vi "hFilterReg2014.vi"(4 "error in":errorcluster, 5 "Filter Modus":u16 format="%x", 6 "Frequenz":u16 format="%x", 7 "FPGA VI Reference In":refnum<k20>) -> (0 "error out":errorcluster, 2 "Timed Out":bool, 3 "FPGA VI Reference Out":refnum<k20>)   [LabVIEW 2014]
doc: "Schreibt eine gemeinsame Konfiguration in alle Filterregister."
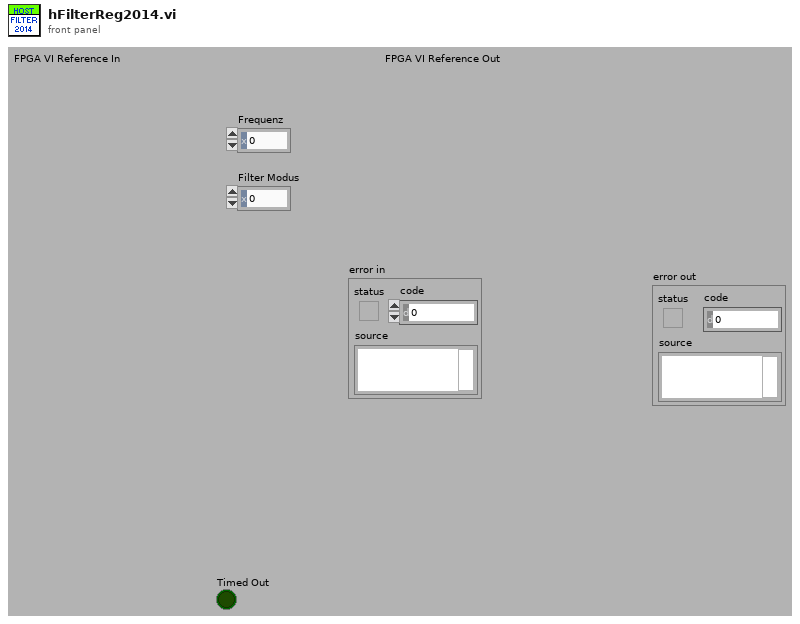
[diagram p1: front panel]
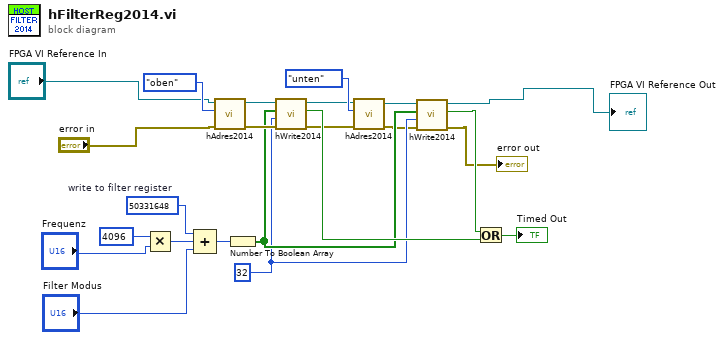
[diagram p0: block diagram]
diagram:
  w20 = u32 50331648  # write to filter register
  w6 = u8 32
  n1 = Multiply(x=u32 4096, y="Frequenz") -> (x*y=w21:u32)
  n2 = Compound Arithmetic op=ADD(w20, w21, "Filter Modus") -> (w22:u32)
  n3 = call "hAdres2014.vi"("error in"="error in", "AdressMode"=enum16{"select", "oben", "unten", "keinen"}."oben", "FPGA VI Reference In"="FPGA VI Reference In") -> ("error out"=w12:errorcluster, "FPGA VI Reference Out"=w13:refnum<k20>)  [unwired: 3 in]
  n4 = Number To Boolean Array(number=w22) -> (Boolean array=w7:bool[])
  n5 = call "hWrite2014.vi"("error in"=w12, "nbit"=w6, "Data"=w7, "FPGA VI Reference In"=w13) -> ("error out"=w9:errorcluster, "Timed Out"=w11:bool, "FPGA VI Reference Out"=w10:refnum<k20>)  [unwired: 1 in]
  n6 = call "hAdres2014.vi"("error in"=w9, "AdressMode"=enum16{"select", "oben", "unten", "keinen"}."unten", "FPGA VI Reference In"=w10) -> ("error out"=w5:errorcluster, "FPGA VI Reference Out"=w8:refnum<k20>)  [unwired: 3 in]
  n7 = call "hWrite2014.vi"("error in"=w5, "nbit"=w6, "Data"=w7, "FPGA VI Reference In"=w8) -> ("error out"=→"error out":errorcluster, "Timed Out"=w3:bool, "FPGA VI Reference Out"=→"FPGA VI Reference Out":refnum<k20>)  [unwired: 1 in]
  n8 = Or(x=w3, y=w11) -> (x .or. y?=→"Timed Out":bool)
